vi "Set Strings from Ref.vi"(8 "error in (no error)":errorcluster, 9 "Language Index (0)":i32, 10 "GObj Refnum":refnum<vi>, 11 "WaveformGraph in":refnum<class "IntensityGraph.lvclass">) -> (0 "error out":errorcluster, 3 "WaveformGraph out":refnum<class "IntensityGraph.lvclass">)   [LabVIEW 2013, in "SET Project Data.lvlib" / "IntensityGraph.lvclass"]
uses:
  IntensityGraph.lvclass
  GraphChart/GraphChart.lvclass
  GObject/GObject.lvclass
  SET Project Data.lvlib
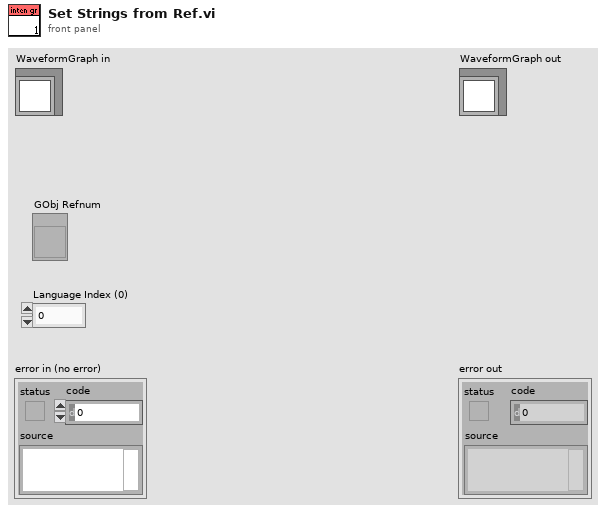
[diagram p1: front panel]
types:
  T1 = typedef "LVCursorListTypeDef.ctl" = cluster{"Name":string, "Color":u32, "Style":u8, "Point Style":u8, "Name Visible":bool, "Allow Drag":bool, "Cursor Mode":u32, "Plot":i32, "Index":i32, "Position":cluster{"X":dbl, "Y":dbl}, "X Scale":u32, "Y Scale":u32, "Watch Plots":i32[], "Watch All Plots":bool, "Plot Area":i32, "Label Offset":cluster{"X":dbl, "Y":dbl}}[]
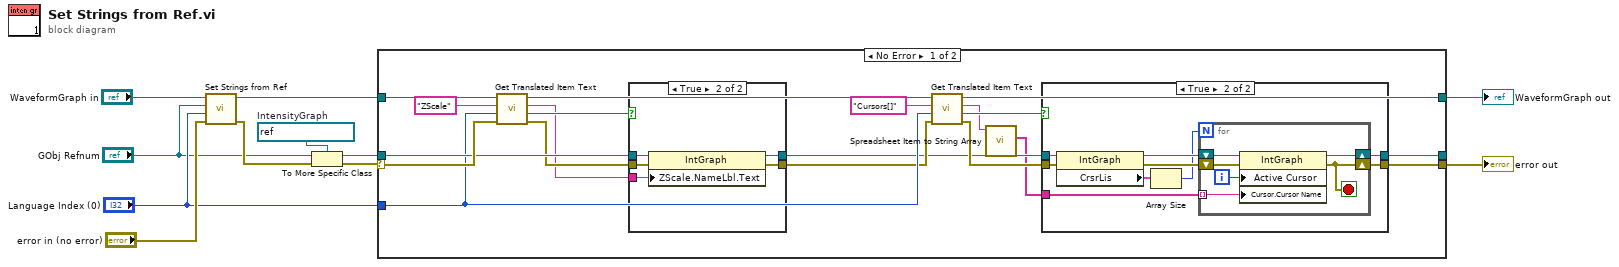
[diagram p0: block diagram]
diagram:
  w7 = refnum<vi> refnum  # IntensityGraph
  n1 = call-parent "Set Strings from Ref.vi"("error in (no error)"="error in (no error)", "Language Index (0)"="Language Index (0)", "GObj Refnum"="GObj Refnum", "GraphChart in"="WaveformGraph in") -> ("error out"=w5:errorcluster, "GraphChart out"=w6:refnum<class "IntensityGraph.lvclass">)  [unwired: 6 in]
  n2 = To More Specific Class(target class=w7, reference="GObj Refnum", error in=w5) -> (specific class reference=w9:refnum<vi>, error out=w8:errorcluster)
  n3 = case shown="No Error" w8 {
    selector: w8 -> [w28 w56]
    tunnel: w9 -> [w26 w55]
    tunnel: w6 -> [w29 w57]
    tunnel: "Language Index (0)" -> [w21 _]
    tunnel: [w17 w57] -> w2
    tunnel: [w14 w56] -> w1
    tunnel: [w13 w55] -> _
    frame No Error {
      n4 = call "Get Translated Item Text.vi"("error in (no error)"=w28, "LangIndex (0)"=w21, "ItemName"="ZScale", "GObject in"=w29) -> ("error out"=w25:errorcluster, "Found?"=w27:bool, "Translated Text (ASCII)"=w12:string, "GObject out"=w23:refnum<class "IntensityGraph.lvclass">)  [unwired: 4 in]
      n5 = case shown="True" w27 {
        tunnel: w26 -> [w48 w54]
        tunnel: w12 -> [_ w51]
        tunnel: w25 -> [w49 w52]
        tunnel: [w49 w50] -> w20
        tunnel: [w48 w53] -> w18
        frame False {
        }
        frame True {
          n6 = property class="IntGraph"(reference=w54, error in=w52, "ZScale.NameLbl.Text"=w51) -> (reference out=w53:refnum<vi>, error out=w50:errorcluster)
        }
      }
      n7 = call "Get Translated Item Text.vi"("error in (no error)"=w20, "LangIndex (0)"=w21, "ItemName"="Cursors[]", "GObject in"=w23) -> ("error out"=w19:errorcluster, "Found?"=w22:bool, "Translated Text (ASCII)"=w16:string, "GObject out"=w17:refnum<class "IntensityGraph.lvclass">)  [unwired: 4 in]
      n8 = call "Spreadsheet Item to String Array.vi"("Spreadsheet Item (ASCII)"=w16) -> ("Strings [] (ASCII)"=w15:string[])  [unwired: 10 in]
      n9 = case shown="True" w22 {
        tunnel: w18 -> [w31 w37]
        tunnel: w15 -> [_ w41]
        tunnel: w19 -> [w32 w36]
        tunnel: [w32 w40] -> w14
        tunnel: [w31 w39] -> w13
        frame False {
        }
        frame True {
          n10 = property class="IntGraph"(reference=w37, error in=w36) -> (reference out=w35:refnum<vi>, error out=w34:errorcluster, "CrsrLis"=w38:T1)
          n11 = Array Size(array=w38) -> (size(s)=w33:i32)
          n12 = for {
            N: w33 -> [_]
            tunnel: w41 -> [w45] mode=indexing
            shift-right: [w44] -> w39
            shift-left: w35 -> [w47]
            shift-right: [w42] -> w40
            shift-left: w34 -> [w43]
            i -> [w46]
            stop <- w42 stop-if-true
            n13 = property class="IntGraph"(reference=w47, error in=w43, "Active Cursor"=w46, "Cursor.Cursor Name"=w45) -> (reference out=w44:refnum<vi>, error out=w42:errorcluster)
          }
        }
      }
    }
    frame Error {
    }
  }
  "error out" <- w1
  "WaveformGraph out" <- w2
